vi "xyBroadcastToDashboardApp.vi"(8 "y":dbl, 11 "x":dbl) -> ()   [LabVIEW 2014]
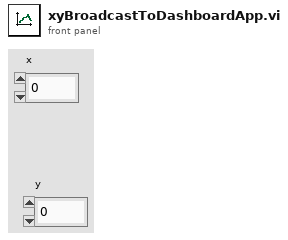
[diagram p1: front panel]
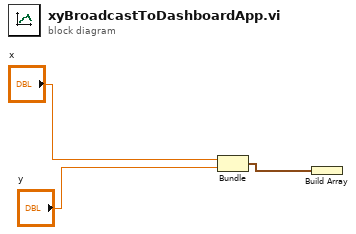
[diagram p0: block diagram]
diagram:
  n1 = Bundle("x"="x", "y"="y") -> (w1:cluster{"x":dbl, "y":dbl})  [unwired: 1 in]
  n2 = Build Array(w1) -> ()  [unwired: 1 out]
